vi "Add Panel.vi"(6 "Events":T1, 7 "Parent":string, 8 "error in (no error)":errorcluster, 10 "Panel":string) -> (0 "error out":errorcluster)   [LabVIEW 2020, in "Panel.lvlib" / "Panel Registry.lvclass"]
doc: "Adds a panel to a parent panel.\n\n----\nPlease see the following web address for additional documentation and tutorial information:\nhttp://www.mooregoodideas.com/mgi-panel-manager/\n\nAuthor: Derek Trepanier\n\nCopyright (c) 2018, Moore Good Ideas, Inc.\n\nAll rights reserved.\n\nRedistribution and use in source and binary forms, with or without modification, are permitted provided that the following conditions are met:\n\n * Redistributions of source code must retain the above copyright notice, this list of conditions and the following disclaimer.\n * Redistributions in binary form must reproduce the above copyright notice, this list of conditions and the following disclaimer in the documentation and/or other materials provided with the distribution.\n * Neither the name of Moore Good Ideas, Inc. nor the names of its contributors may be used to endorse or promote products derived from this software without specific prior written permission.\n\nTHIS SOFTWARE IS PROVIDED BY THE COPYRIGHT HOLDERS AND CONTRIBUTORS \"AS IS\" AND ANY EXPRESS OR IMPLIED WARRANTIES, INCLUDING, BUT NOT LIMITED TO, THE IMPLIED WARRANTIES OF MERCHANTABILITY AND FITNESS FOR A PARTICULAR PURPOSE ARE DISCLAIMED. IN NO EVENT SHALL THE COPYRIGHT OWNER OR CONTRIBUTORS BE LIABLE FOR ANY DIRECT, INDIRECT, INCIDENTAL, SPECIAL, EXEMPLARY, OR CONSEQUENTIAL DAMAGES (INCLUDING, BUT NOT LIMITED TO, PROCUREMENT OF SUBSTITUTE GOODS OR SERVICES; LOSS OF USE, DATA, OR PROFITS; OR BUSINESS INTERRUPTION) HOWEVER CAUSED AND ON ANY THEORY OF LIABILITY, WHETHER IN CONTRACT, STRICT LIABILITY, OR TORT (INCLUDING NEGLIGENCE OR OTHERWISE) ARISING IN ANY WAY OUT OF THE USE OF THIS SOFTWARE, EVEN IF ADVISED OF THE POSSIBILITY OF SUCH DAMAGE."
uses:
  <vilib>/MGI/Panel Manager/Panel/Panel Registry/Panel Registry.lvclass
  <vilib>/MGI/Panel Manager/Panel/Panel Helper/Panel Events.ctl
  <vilib>/MGI/Panel Manager/Panel/Panel Helper/Events.ctl
  <vilib>/MGI/Panel Manager/Panel/Panel Registry/Panel Registry.lvclass/Panel Registry.ctl
  <vilib>/MGI/Panel Manager/Panel/Cursor/Lookup Actions.ctl
  <vilib>/MGI/Panel Manager/Panel/Panel Helper/Panel Helper.lvclass
  <vilib>/MGI/Panel Manager/Panel/Cursor/Cursor.lvclass
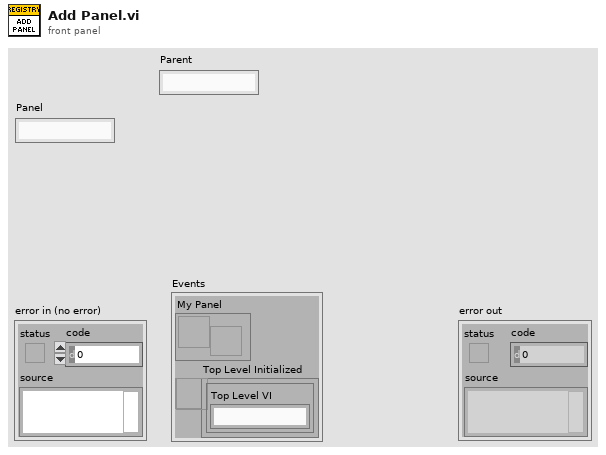
[diagram p1: front panel]
types:
  T1 = typedef "Panel.lvlib/Panel Helper.lvclass/Panel Events.ctl" = cluster{"My Panel":refnum<user-event>, "Top Level Initialized":refnum<user-event>}
  T2 = typedef "Panel.lvlib/Panel Helper.lvclass/Events.ctl" = enum16{"Initialized", "Shown", "Hidden", "Closed"}
  T3 = typedef "Panel.lvlib/Cursor.lvclass/Lookup Actions.ctl" = enum16{"Init", "Get", "Destroy"}
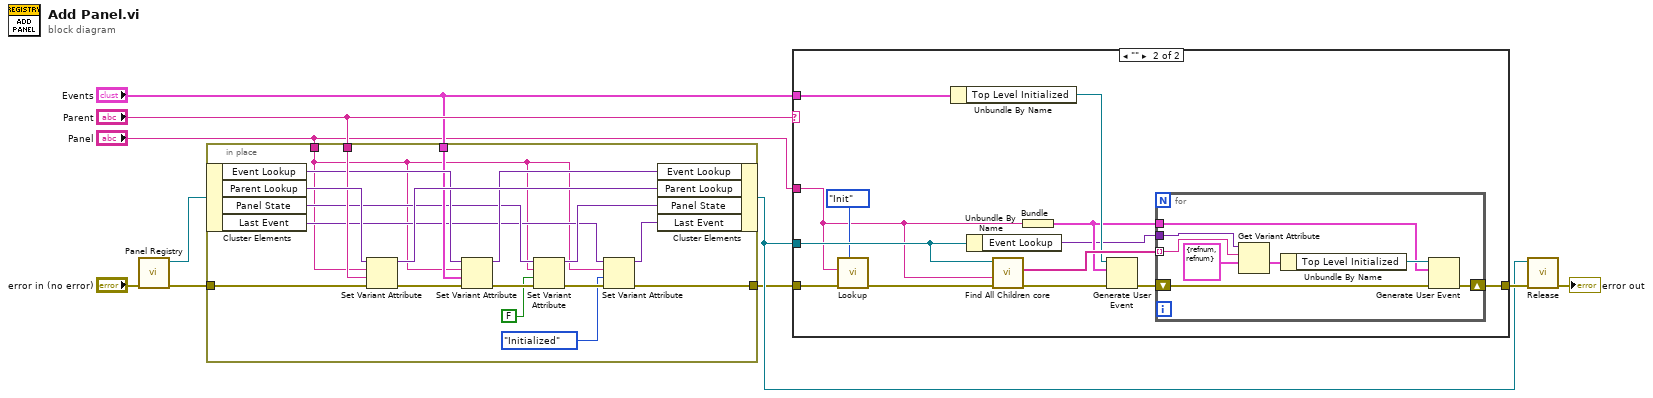
[diagram p0: block diagram]
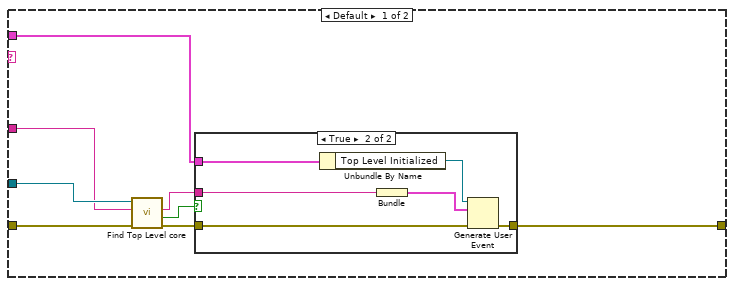
[diagram p2: hidden frame]
diagram:
  n1 = call <vilib>:"Panel Registry.vi"("error in (no error)"="error in (no error)") -> ("error out"=w4:errorcluster, "Panel Registry out"=w8:refnum<class "Panel Registry.lvclass">)  [unwired: 9 in]
  n2 = in-place {
    in-place-border: "Panel" -> [w13]
    in-place-border: "Parent" -> [w27]
    in-place-border: "Events" -> [w23]
    in-place-border: w4 -> [w22]
    in-place-border: [w11] -> w3
    n3 = in-place-cluster #1(w8) -> ("Event Lookup"=w25:variant, "Parent Lookup"=w28:variant, "Panel State"=w18:variant, "Last Event"=w15:variant)
    n4 = Set Variant Attribute(Variant=w28, name=w13, value=w27, error in=w22) -> (Variant out=w26:variant, error out=w21:errorcluster)  [unwired: 1 out]
    n5 = Set Variant Attribute(Variant=w25, name=w13, value=w23, error in=w21) -> (Variant out=w24:variant, error out=w20:errorcluster)  [unwired: 1 out]
    n6 = Set Variant Attribute(Variant=w18, name=w13, value=FALSE, error in=w20) -> (Variant out=w19:variant, error out=w16:errorcluster)  [unwired: 1 out]
    n7 = Set Variant Attribute(Variant=w15, name=w13, value=Events."Initialized" ("Event"), error in=w16) -> (Variant out=w14:variant, error out=w11:errorcluster)  [unwired: 1 out]
    n8 = in-place-cluster #1("Event Lookup"=w24, "Parent Lookup"=w26, "Panel State"=w19, "Last Event"=w14) -> (w5:refnum<class "Panel Registry.lvclass">)
  }
  n9 = case shown="\"\"" "Parent" {
    tunnel: [w35 w55] -> w9
    tunnel: w3 -> [w34 w46]
    tunnel: "Panel" -> [w29 w44]
    tunnel: "Events" -> [w36 w54]
    tunnel: w5 -> [w32 w49]
    frame Default {
      n10 = call <vilib>:"Find Top Level core.vi"("error in (no error)"=w34, "VI"=w29, "Panel Registry in"=w32) -> ("error out"=w33:errorcluster, "Found?"=w30:bool, "Top Level Panel"=w31:string)  [unwired: 6 in]
      n11 = case shown="True" w30 {
        tunnel: w36 -> [_ w43]
        tunnel: w31 -> [_ w41]
        tunnel: w33 -> [w37 w39]
        tunnel: [w37 w38] -> w35
        frame False {
          # "Top Level not yet initialized"
        }
        frame True {
          n12 = Unbundle By Name(w43) -> ("Top Level Initialized"=w42:refnum<user-event>)
          n13 = Bundle("Top Level Panel"=w41) -> (w40:cluster{"Top Level Panel":string})  [unwired: 1 in]
          n14 = Generate User Event(user event=w42, event data cluster=w40, error in=w39) -> (error out=w38:errorcluster)  [unwired: 1 in, 1 out]
        }
      }
    }
    frame "" {
      n15 = call <vilib>:"Lookup.vi"("Action"=Lookup_Actions."Init", "error in (no error)"=w46, "Top Level VI"=w44) -> ("error out"=w45:errorcluster)  [unwired: 7 in, 1 out]
      n16 = Unbundle By Name(w54) -> ("Top Level Initialized"=w53:refnum<user-event>)
      n17 = Unbundle By Name(w49) -> ("Event Lookup"=w48:variant)
      n18 = call <vilib>:"Find All Children core.vi"("error in (no error)"=w45, "Panel"=w44, "Panel Registry in"=w49) -> ("error out"=w51:errorcluster, "All Children"=w56:string[])  [unwired: 7 in]
      n19 = Bundle("Panel"=w44) -> (w52:cluster{"Panel":string})  [unwired: 1 in]
      n20 = Generate User Event(user event=w53, event data cluster=w52, error in=w51) -> (error out=w50:errorcluster)  [unwired: 1 in, 1 out]
      n21 = for {
        shift-right: [w57] -> w55
        shift-left: w50 -> [w58]
        tunnel: w56 -> [w63] mode=indexing
        tunnel: w48 -> [w64]
        tunnel: w52 -> [w59]
        n22 = Get Variant Attribute(Variant=w64, name=w63, default value (empty Variant)=T1 {"My Panel"=refnum, "Top Level Initialized"=refnum} ("Events")) -> (value=w61:T1)  [unwired: 1 in, 3 out]
        n23 = Unbundle By Name(w61) -> ("Top Level Initialized"=w60:refnum<user-event>)
        n24 = Generate User Event(user event=w60, event data cluster=w59, error in=w58) -> (error out=w57:errorcluster)  [unwired: 1 in, 1 out]
      }
    }
  }
  n25 = call <vilib>:"Release.vi"("error in (no error)"=w9, "Panel Registry in"=w5) -> ("error out"=→"error out":errorcluster)  [unwired: 9 in]
